vi "main.vi"() -> ()   [LabVIEW 2013]
uses:
  <vilib>/Analysis/baseanly.llb/Mean (DBL).vi
  major_subprograms/turn_off_global_variable.vi
  <vilib>/Analysis/NI_AALBase.lvlib
panel:
  in  "Traces to show":i32=10
  out "Million samples":dbl=63.998
  out "Readout time (s)":dbl=0.019999375
  out "Done":bool=TRUE
  out "Number of records":i32=31999
  out "Channel A":i16[][](graph)
  out "Squares":dbl[][](graph)
  out "Channel B":i16[][](graph)
  in  "Stop the safe way":bool
  out "Samples per run":i16=2000
  in  "Tab Control":enum32{"Setup", "Data collection", "Saving"}(tab)=enum."Data collection"
  in  "Blink?":bool
  in  "Trigger":enum32{"Software", "Level", "External"}(radio)=enum."External"
  in  "Number of records":u16(ring)=1 items=["Maximal", "User-defined"]
  in  "Pulse interval (ns)":i16=1000 min=1
  in  "Number of pulses":i16=5 min=1
  in  "Number of records 2":i16=1000 min=1
  in  "Save Squares?":bool
  in  "fileName":string="data_labview_"
  # "Number of pulses"
  # "Trigger\nHere"
  # "Pulse interval"
  # "One run"
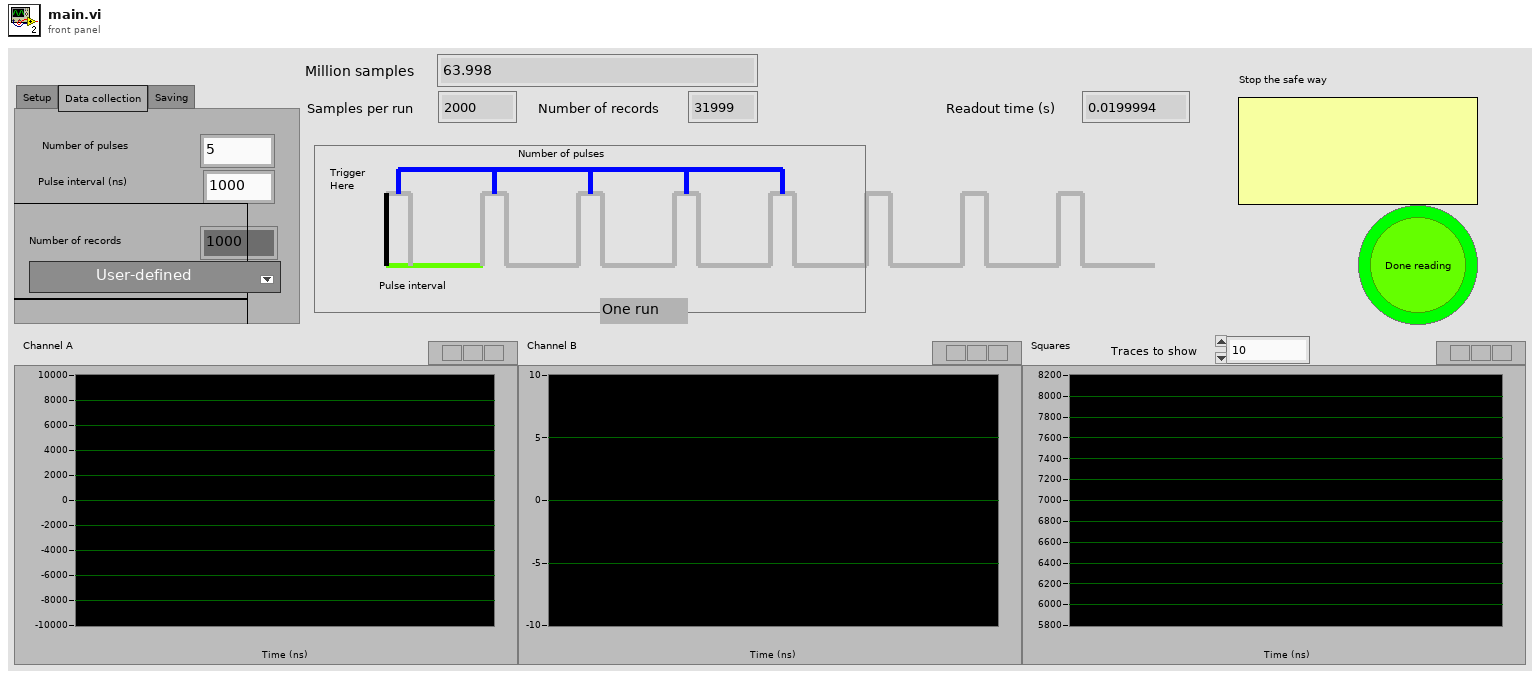
[diagram p1: front panel]
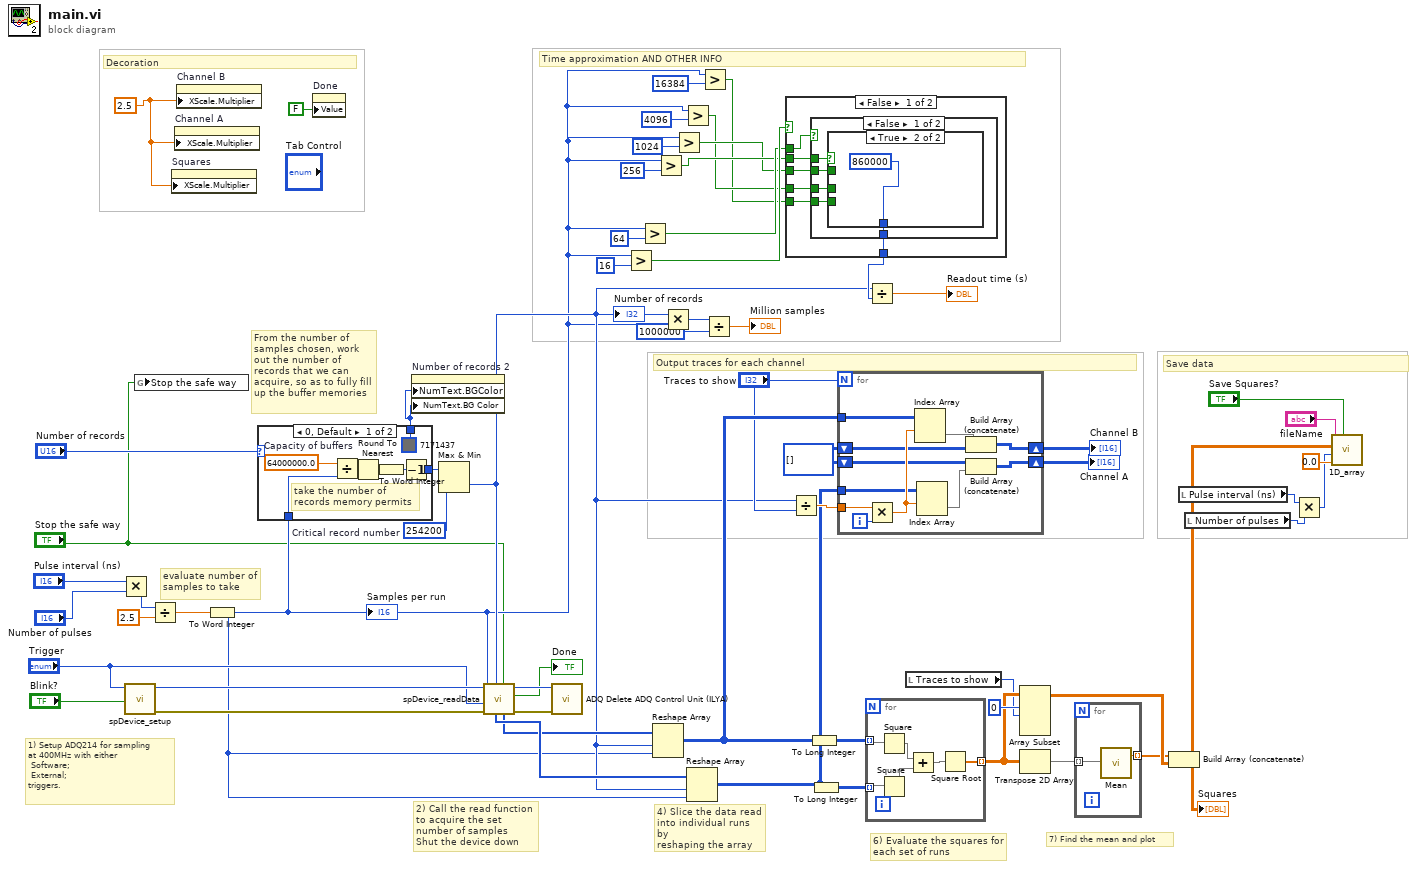
[diagram p0: block diagram]
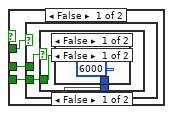
[diagram p2: hidden frame]
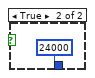
[diagram p3: hidden frame]
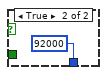
[diagram p4: hidden frame]
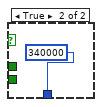
[diagram p5: hidden frame]
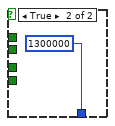
[diagram p6: hidden frame]
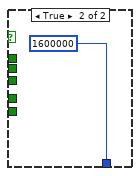
[diagram p7: hidden frame]
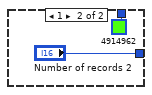
[diagram p8: hidden frame]
diagram:
  w35 = 254200  # Critical record number
  w45 = 2.5 ("X Scale.Offset and Multiplier:Multiplier")
  w51 = i16[][] []
  # "Save data"
  # "Decoration"
  # "Time approximation AND OTHER INFO"
  # "From the number of samples chosen, work out the number of records that we can acquire, so as to fully fill up the buffer memories"
  # "evaluate number of samples to take"
  # "7) Find the mean and plot"
  # "6) Evaluate the squares for\neach set of runs"
  # "Output traces for each channel"
  # "4) Slice the data read into individual runs by\nreshaping the array"
  # "2) Call the read function to acquire the set\nnumber of samples\nShut the device down"
  # "1) Setup ADQ214 for sampling\nat 400MHz with either\n Software;\n External;\ntriggers."
  n1 = Multiply(x="Pulse interval (ns)", y="Number of pulses") -> (x*y=w57:i16)
  n2 = call "spDevice_setup.vi"("Blink?"="Blink?", "Trigger"="Trigger") -> ("error out"=w61:errorcluster, "adq_cu_ptr"=w62:u32)  [unwired: 6 in, 2 out]
  n3 = global write "turn_off_global_variable.vi" "Stop the safe way"("Stop the safe way") -> ()
  n4 = Divide(x=w57, y=sgl 2.5) -> (x/y=w55:sgl)
  n5 = property on="Squares" class="WFGraph (strict)"("XScale.Multiplier"=w45) -> ()  [unwired: 2 in, 2 out]
  n6 = property on="Channel A" class="WFGraph (strict)"("XScale.Multiplier"=w45) -> ()  [unwired: 2 in, 2 out]
  n7 = property on="Channel B" class="WFGraph (strict)"("XScale.Multiplier"=w45) -> ()  [unwired: 2 in, 2 out]
  n8 = To Word Integer(number=w55) -> (16bit integer=w15:i16)
  "Samples per run" <- w15
  n9 = case shown="0, Default" "Number of records" {
    tunnel: w15 -> [w65 _]
    tunnel: [u32 7171437 u32 4914962] -> w31
    tunnel: [w63 "Number of records 2"] -> w2
    frame 0, Default {
      w68 = 64000000.0  # Capacity of buffers
      # "take the number of records memory permits"
      n10 = Divide(x=w68, y=w65) -> (x/y=w69:dbl)
      n11 = Round To Nearest(number=w69) -> (nearest integer value=w66:dbl)
      n12 = To Word Integer(number=w66) -> (16bit integer=w67:i16)
      n13 = Decrement(x=w67) -> (x-1=w63:i16)
    }
    frame 1 {
    }
  }
  n14 = property on="Done" class="Bool (strict)"("Value"=FALSE ("Done reading")) -> ()  [unwired: 2 in, 2 out]
  n15 = property on="Number of records 2" class="DigNum (strict)"("NumText.BGColor"=w31, "NumText.BG Color"=w31) -> ()  [unwired: 2 in, 2 out]
  n16 = Max & Min(x=w2, y=w35) -> (min(x,y)=w16:i32)  [unwired: 1 out]
  "Number of records" <- w16
  n17 = call "spDevice_readData.vi"("Dont wait"="Stop the safe way", "Number of records"=w16, "error in (no error)"=w61, "Trigger"="Trigger", "Samples per record"=w15, "adq_cu_ptr in"=w62) -> ("error out"=w60:errorcluster, "Done reading"=→"Done":bool, "adq_cu_ptr out"=w59:u32, "buffer_chB_out"=w53:i16[], "buffer_chA_out"=w54:i16[])  [unwired: 1 in]
  n18 = call "ADQ Delete ADQ Control Unit (ILYA).vi"("error in (no error)"=w60, "adq_cu_ptr"=w59) -> ()  [unwired: 7 in, 3 out]
  n19 = Greater?(x=w15, y=16) -> (0:w24:bool)
  n20 = Greater?(x=w15, y=64) -> (0:w23:bool)
  n21 = Reshape Array(w53, w16, w15) -> (w49:i16[][])
  n22 = Greater?(x=w15, y=256) -> (0:w22:bool)
  n23 = Multiply(x=w16, y=w15) -> (x*y=w14:i32)
  n24 = Greater?(x=w15, y=1024) -> (0:w21:bool)
  n25 = Greater?(x=w15, y=4096) -> (0:w20:bool)
  n26 = Reshape Array(w54, w16, w15) -> (w48:i16[][])
  n27 = Greater?(x=w15, y=16384) -> (0:w19:bool)
  n28 = Divide(x=w14, y=1000000) -> (x/y=→"Million samples":dbl)
  n29 = case shown="False" w24 {
    tunnel: [w76 1600000 ("y")] -> w18
    tunnel: w23 -> [w77 _]
    tunnel: w22 -> [w75 _]
    tunnel: w21 -> [w74 _]
    tunnel: w20 -> [w73 _]
    tunnel: w19 -> [w72 _]
    frame False {
      n30 = case shown="False" w77 {
        tunnel: [w81 1300000 ("y")] -> w76
        tunnel: w75 -> [w82 _]
        tunnel: w74 -> [w80 _]
        tunnel: w73 -> [w79 _]
        tunnel: w72 -> [w78 _]
        frame False {
          n31 = case shown="True" w82 {
            tunnel: [w85 860000 ("y")] -> w81
            tunnel: w80 -> [w86 _]
            tunnel: w79 -> [w84 _]
            tunnel: w78 -> [w83 _]
            frame False {
              n32 = case shown="False" w86 {
                tunnel: [w88 340000 ("y")] -> w85
                tunnel: w84 -> [w89 _]
                tunnel: w83 -> [w87 _]
                frame False {
                  n33 = case shown="False" w89 {
                    tunnel: [w90 92000 ("y")] -> w88
                    tunnel: w87 -> [w91 _]
                    frame False {
                      n34 = case shown="False" w91 {
                        tunnel: [6000 ("y") 24000 ("y")] -> w90
                        frame False {
                        }
                        frame True {
                        }
                      }
                    }
                    frame True {
                    }
                  }
                }
                frame True {
                }
              }
            }
            frame True {
            }
          }
        }
        frame True {
        }
      }
    }
    frame True {
    }
  }
  n35 = Divide(x=w16, y="Traces to show") -> (x/y=w52:dbl)
  n36 = To Long Integer(number=w49) -> (32bit integer=w46:i32[][])
  n37 = To Long Integer(number=w48) -> (32bit integer=w47:i32[][])
  n38 = for {
    N: "Traces to show" -> [_]
    tunnel: w49 -> [w105]
    tunnel: w48 -> [w106]
    tunnel: w52 -> [w108]
    shift-right: [w103] -> w43
    shift-left: w51 -> [w102]
    shift-right: [w100] -> w44
    shift-left: w51 -> [w99]
    i -> [w109]
    n39 = Multiply(x=w108, y=w109) -> (x*y=w107:dbl)
    n40 = Index Array(array=w105, index (row)=w107) -> (element=w104:i16[])  [unwired: 1 in]
    n41 = Index Array(array=w106, index (row)=w107) -> (element=w101:i16[])  [unwired: 1 in]
    n42 = Build Array (concatenate)(w104, w102) -> (w103:i16[][])
    n43 = Build Array (concatenate)(w99, w101) -> (w100:i16[][])
  }
  "Channel B" <- w43
  "Channel A" <- w44
  n44 = for {
    tunnel: w46 -> [w115] mode=indexing
    tunnel: [w110] -> w41 mode=indexing
    tunnel: w47 -> [w114] mode=indexing
    n45 = Square(x=w115) -> (x^2=w113:i32[])
    n46 = Square(x=w114) -> (x^2=w112:i32[])
    n47 = Add(x=w113, y=w112) -> (x+y=w111:i32[])
    n48 = Square Root(x=w111) -> (sqrt(x)=w110:dbl[])
  }
  n49 = Divide(x=w16, y=w18) -> (x/y=→"Readout time (s)":dbl)
  n50 = local read "Traces to show"() -> (w3:i32)
  n51 = Array Subset(array=w41, index (row)=0 ("index"), length (row)=w3) -> (w39:dbl[][])  [unwired: 2 in]
  n52 = Transpose 2D Array(2D array=w41) -> (transposed array=w40:dbl[][])
  n53 = for {
    tunnel: w40 -> [w117] mode=indexing
    tunnel: [w116] -> w11 mode=indexing
    n54 = call-poly <vilib>:"Mean.vi"("X"=w117) -> ("mean"=w116:dbl)  [unwired: 1 out]
  }
  n55 = Build Array (concatenate)(w11, w39) -> (w10:dbl[][])
  "Squares" <- w10
  n56 = local read "Pulse interval (ns)"() -> (w9:i16)
  n57 = local read "Number of pulses"() -> (w8:i16)
  n58 = Multiply(x=w9, y=w8) -> (x*y=w4:i16)
  n59 = call "1D_array.vi"("Name"="fileName", "Array"=w10, "x_max"=w4, "x_min"=0.0, "Save?"="Save Squares?") -> ()  [unwired: 1 out]
